vi "Write Data_Coils.vi"(8 "error in (no error)":errorcluster, 9 "register values":bool[](array[boolean]), 11 "Device in":refnum<class "MB_TCP_Device.lvclass">) -> (0 "error out":errorcluster, 3 "Device out":refnum<class "MB_TCP_Device.lvclass">)   [LabVIEW 2023, in "MB_TCP_Device.lvclass"]
uses:
  MB_TCP_Device.lvclass
  MB_TCP_Device.lvclass/MB_TCP_Device.ctl
  <vilib>/NI Modbus.llb/MB Ethernet Master Query Write Multiple Coils (poly).vi
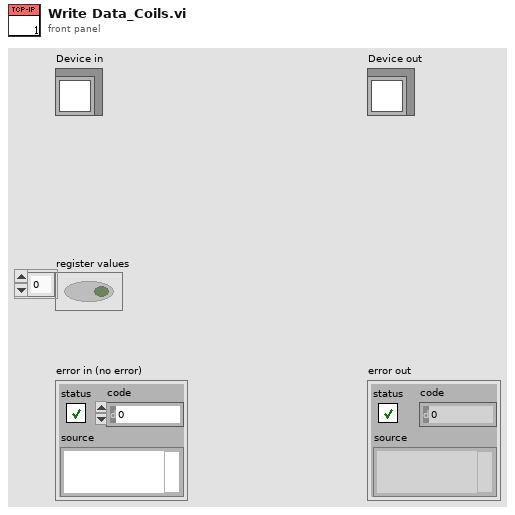
[diagram p1: front panel]
types:
  T1 = typedef "DAQ Device_IO ChannelsData.ctl" = cluster{"#DigitalInputs":u16, "StartAddress_DI":u16, "#DigitalOutputs":u16, "StartAddress_DO":u16, "#AnalogInputs":u16, "StartAddress_AI":u16, "#AnalogOutputs":u16, "StartAddress_AO":u16, "Coil_ReadData":bool[], "Coil_WriteData":bool[], "AI_Data":u16[], "AO_Data":u16[]}
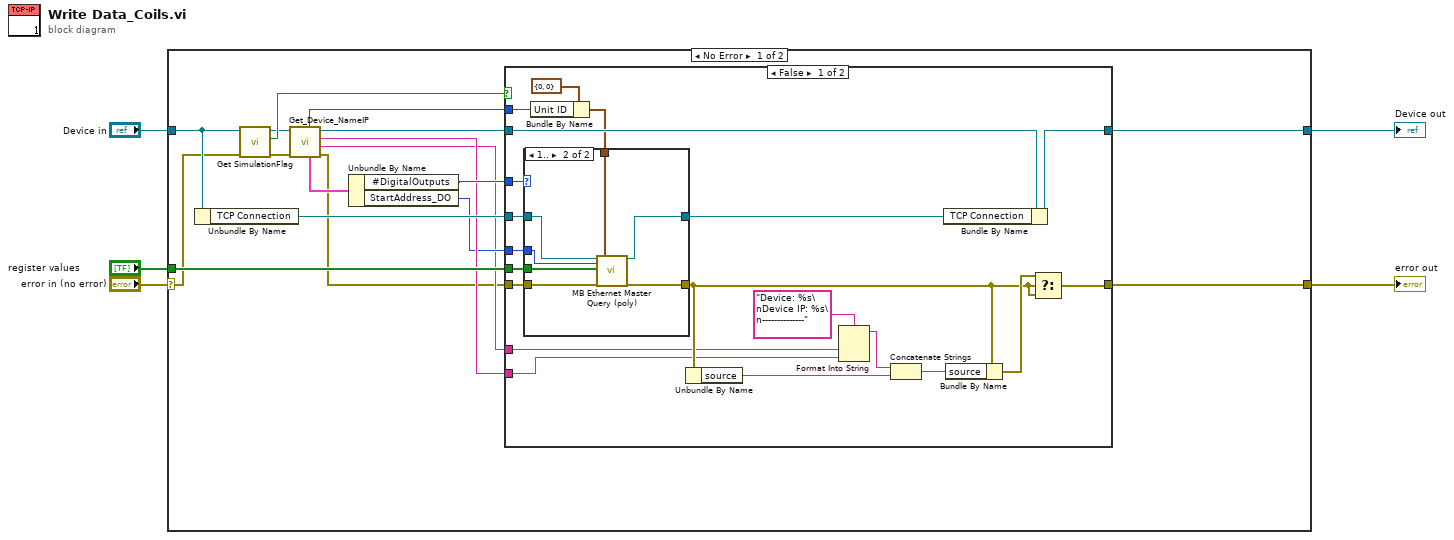
[diagram p0: block diagram]
diagram:
  n1 = case shown="No Error" "error in (no error)" {
    selector: "error in (no error)" -> [w7 w55]
    tunnel: [w20 w55] -> w4
    tunnel: [w22 w54] -> w2
    tunnel: "Device in" -> [w18 w54]
    tunnel: "register values" -> [w21 _]
    frame No Error {
      n2 = Unbundle By Name(w18) -> ("TCP Connection"=w19:refnum<k5>)
      n3 = call-dynamic "Get SimulationFlag.vi"("error in (no error)"=w7, "Device in"=w18) -> ("error out"=w8:errorcluster, "Simulation?"=w17:bool, "Device out"=w16:refnum<class "MB_TCP_Device.lvclass">)  [unwired: 7 in]
      n4 = call-dynamic "Get_Device_NameIP.vi"("error in (no error)"=w8, "Device in"=w16) -> ("error out"=w6:errorcluster, "Device Name"=w10:string, "Device Address"=w12:string, "Device out"=w15:refnum<class "MB_TCP_Device.lvclass">, "IO Channels"=w14:T1, "Unit ID"=w9:u8)  [unwired: 4 in]
      n5 = Unbundle By Name(w14) -> ("#DigitalOutputs"=w13:u16, "StartAddress_DO"=w11:u16)
      n6 = case shown="False" w17 {
        tunnel: [w42 w53] -> w22
        tunnel: w6 -> [w40 w52]
        tunnel: w11 -> [w39 _]
        tunnel: w21 -> [w27 _]
        tunnel: [w36 w52] -> w20
        tunnel: w19 -> [w35 _]
        tunnel: w12 -> [w33 _]
        tunnel: w15 -> [w31 w53]
        tunnel: w10 -> [w30 _]
        tunnel: w13 -> [w26 _]
        tunnel: w9 -> [w23 _]
        frame False {
          n7 = Bundle By Name(cluster=cluster{"Transaction ID":u16, "Unit ID":u8} {"Transaction ID"=0, "Unit ID"=0} ("MBAP Header"), "Unit ID"=w23) -> (w24:cluster{"Transaction ID":u16, "Unit ID":u8})
          n8 = case shown="1.." w26 {
            tunnel: [w44 w51] -> w41
            tunnel: w40 -> [w43 w50]
            tunnel: w39 -> [_ w49]
            tunnel: [w43 w48] -> w37
            tunnel: w35 -> [w44 w47]
            tunnel: w27 -> [_ w46]
            tunnel: w24 -> [_ w45]
            frame 0, Default {
            }
            frame 1.. {
              n9 = call-poly <vilib>:"MB Ethernet Master Query (poly).vi"("TCP Connection Refnum in"=w47, "Starting Address"=w49, "Coils"=w46, "error in"=w50, "MBAP Header"=w45) -> ("TCP Connection Refnum (dup)"=w51:refnum<k5>, "error out"=w48:errorcluster)  [unwired: 12 in, 1 out]
            }
          }
          n10 = Unbundle By Name(w37) -> ("source"=w34:string)
          n11 = Format Into String(format string="Device: %s\nDevice IP: %s\n--------------", w30, w33) -> (resulting string=w29:string)  [unwired: 2 in, 1 out]
          n12 = Concatenate Strings(w29, w34) -> (w28:string)
          n13 = Bundle By Name(cluster=w31, "TCP Connection"=w41) -> (w42:refnum<class "MB_TCP_Device.lvclass">)
          n14 = Bundle By Name(cluster=w37, "source"=w28) -> (w38:errorcluster)
          n15 = Select(t=w38, s=w37, f=w37) -> (s? t:f=w36:errorcluster)
        }
        frame True {
        }
      }
    }
    frame Error {
    }
  }
  "error out" <- w4
  "Device out" <- w2
